vi "DSF.Engine.Plugin.Transfer Group.Build.vi"(8 "error in (no error)":errorcluster, 10 "Transfer Group in":refnum<class "DSF.Engine.Transfer Group.lvclass">, 11 "Plugin in":refnum<class "Plugin.lvclass">) -> (0 "error out":errorcluster, 2 "Transfer Group out":refnum<class "DSF.Engine.Transfer Group.lvclass">, 3 "Plugin out":refnum<class "Plugin.lvclass">)   [LabVIEW 2017, in "DSF.Engine.lvlib" / "Plugin.lvclass"]
uses:
  Plugin.lvclass
  Transfer/DSF.Engine.Transfer Group.lvclass
  Transfer/DSF.Engine.Transfer Group.lvclass/DSF.Engine.Transfer Group.ctl
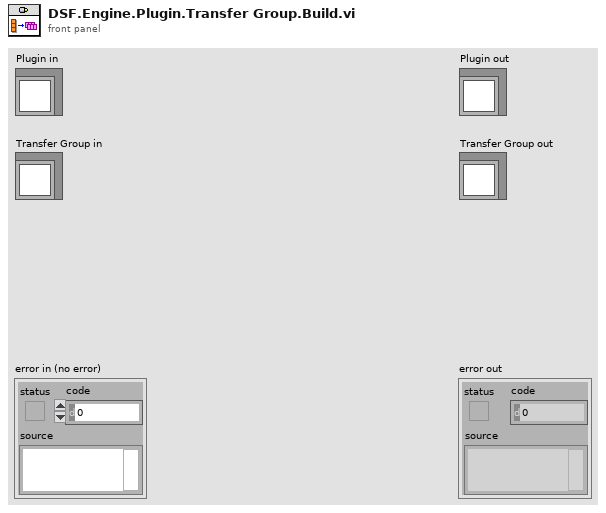
[diagram p1: front panel]
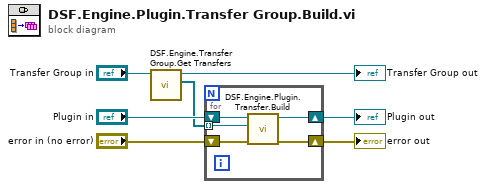
[diagram p0: block diagram]
diagram:
  n1 = call "DSF.Engine.Transfer Group.Get Transfers.vi"("Transfer Group in"="Transfer Group in") -> ("Transfers"=w5:refnum<class "DSF.Engine.Transfer.lvclass">[], "Transfer Group out"=→"Transfer Group out":refnum<class "DSF.Engine.Transfer Group.lvclass">)  [unwired: 9 in]
  n2 = for {
    tunnel: w5 -> [w8] mode=indexing
    shift-right: [w9] -> w4
    shift-left: "Plugin in" -> [w10]
    shift-right: [w11] -> w3
    shift-left: "error in (no error)" -> [w12]
    n3 = call "DSF.Engine.Plugin.Transfer.Build.vi"("error in (no error)"=w12, "Transfer"=w8, "Plugin in"=w10) -> ("error out"=w11:errorcluster, "Plugin out"=w9:refnum<class "Plugin.lvclass">)  [unwired: 7 in]
  }
  "error out" <- w3
  "Plugin out" <- w4
